vi "Fin_clear.vi"(8 "Error In":errorcluster, 11 "Fin Arrangement (SORTED)":u8[](array[numeric])) -> (0 "Error Out":errorcluster)   [LabVIEW 2013]
uses:
  My Computer/Controls/Fin Status.ctl
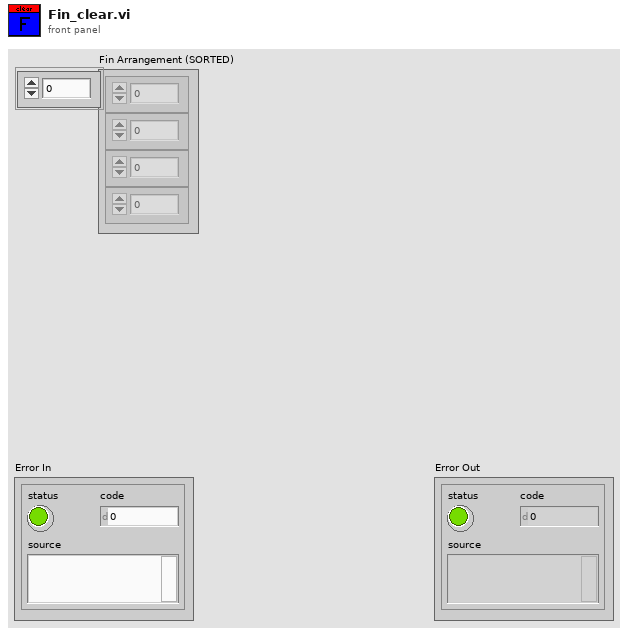
[diagram p1: front panel]
types:
  T1 = typedef "Fin Status.ctl" = u32[]
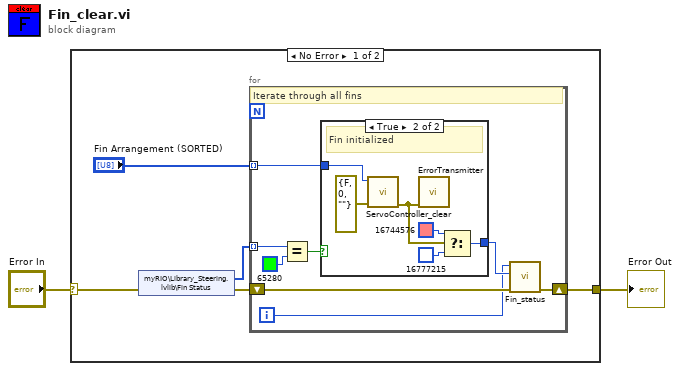
[diagram p0: block diagram]
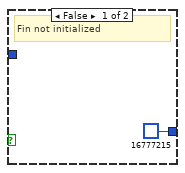
[diagram p2: hidden frame]
diagram:
  n1 = case shown="No Error" "Error In" {
    selector: "Error In" -> [w5 w23]
    tunnel: [w3 w23] -> w1
    frame No Error {
      n2 = shared-variable "myRIO\\Library_Steering.lvlib\\Fin Status"(error in=w5) -> (w7:T1, error out=w4:errorcluster)
      n3 = for {
        tunnel: w7 -> [w14] mode=indexing
        tunnel: "Fin Arrangement (SORTED)" -> [w12] mode=indexing
        shift-right: [w11] -> w3
        shift-left: w4 -> [w10]
        i -> [w8]
        # "Iterate through all fins"
        n4 = Equal?(x=w14, y=u32 65280 ("Round Color Box")) -> (x = y?=w13:bool)
        n5 = case shown="True" w13 {
          tunnel: w12 -> [_ w22]
          tunnel: [u32 16777215 ("Round Color Box") w18] -> w9
          frame False {
            # "Fin not initialized"
          }
          frame True {
            # "Fin initialized"
            n6 = call "ServoController_clear.vi"("Error In"=errorcluster {"status"=FALSE, "code"=0, "source"=""}, "Servo Controller Index"=w22) -> ("Error Out"=w17:errorcluster)  [unwired: 9 in]
            n7 = call "ErrorTransmitter.vi"("Error In"=w17) -> ()  [unwired: 10 in, 1 out]
            n8 = Select(t=u32 16744576 ("Round Color Box"), s=w17, f=u32 16777215 ("Round Color Box")) -> (s? t:f=w18:u32)
          }
        }
        n9 = call "Fin_status.vi"("Error In"=w10, "Round Color Box"=w9, "Fin Index"=w8) -> ("Error Out"=w11:errorcluster)  [unwired: 8 in]
      }
    }
    frame Error {
    }
  }
  "Error Out" <- w1
